vi "FIRE_WHEN_READY.vi"(10 "argv":string[](array[string]), 11 "args":u8) -> ()   [LabVIEW 2011]
uses:
  <vilib>/Rock Robotics/WPI/DriverStation/WPI_DriverStationStatusErrorCache.ctl
  signals/Signal.ctl
  Auto_Conf.vi
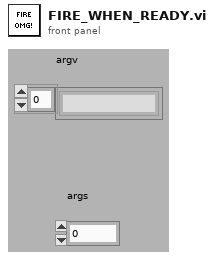
[diagram p1: front panel]
types:
  T1 = typedef "WPI_DriverStationStatusErrorCache.ctl" = enum16{"Get", "Set"}
  T2 = typedef "Signal.ctl" = enum16{"SIGFIRE", "SIGSTOPSCRIPT", "SIGSTARTGUN", "SIGSTOPGUN", "SIGDISABLED", "SIGENABLED", "SIGUDPTIMEOUT", "SIGNEWVISION_REMOTE", "SIGNEWVISION_LOCAL", "SIGSHOTFIRED", "SIGDOTRACK", "SIGDONTTRACK"}
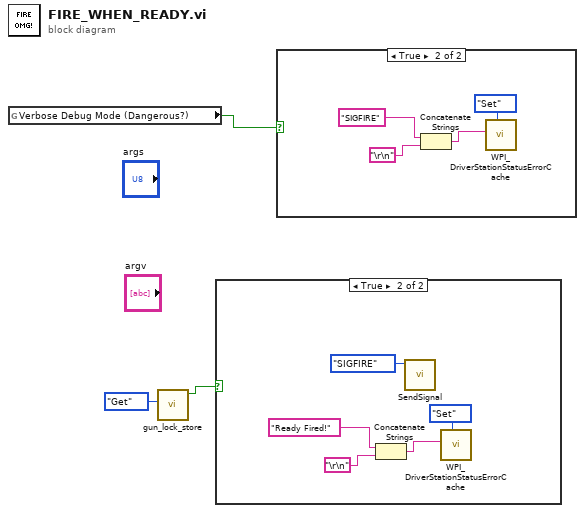
[diagram p0: block diagram]
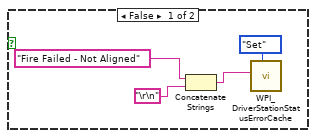
[diagram p2: hidden frame]
diagram:
  n1 = global read "Auto_Conf.vi" "Verbose Debug Mode (Dangerous?)"() -> (w3:bool)
  n2 = call "gun_lock_store.vi"("data_store_mode"=enum16{"Set", "Get"}."Get") -> ("Lock"=w1:bool)  [unwired: 10 in]
  n3 = case shown="True" w1 {
    frame False {
      n4 = Concatenate Strings("Fire Failed - Not Aligned" ("string"), "\r\n") -> (w5:string)
      n5 = call <vilib>:"WPI_DriverStationStatusErrorCache.vi"("StatusErrorCacheOp"=WPI_DriverStationStatusErrorCache."Set", "Error String"=w5) -> ()  [unwired: 10 out]
    }
    frame True {
      n6 = Concatenate Strings("Ready Fired!" ("string"), "\r\n") -> (w10:string)
      n7 = call "SendSignal.vi"("Signal"=Signal."SIGFIRE") -> ()  [unwired: 11 in]
      n8 = call <vilib>:"WPI_DriverStationStatusErrorCache.vi"("StatusErrorCacheOp"=WPI_DriverStationStatusErrorCache."Set", "Error String"=w10) -> ()  [unwired: 10 out]
    }
  }
  n9 = case shown="True" w3 {
    frame False {
    }
    frame True {
      n10 = Concatenate Strings("SIGFIRE" ("string"), "\r\n") -> (w14:string)
      n11 = call <vilib>:"WPI_DriverStationStatusErrorCache.vi"("StatusErrorCacheOp"=WPI_DriverStationStatusErrorCache."Set", "Error String"=w14) -> ()  [unwired: 10 out]
    }
  }
